vi "Configure Math Function (Low-pass).vi"(4 "Math Function Index (1: Math Function 1)":i32(ring)=1 items=["Math Function 1"=1, "Math Function 2"=2, "Math Function 3"=3, "Math Function 4"=4], 8 "error in (no error)":errorcluster, 10 "Low-Pass Frequency (1E+9)":dbl=1000000000.0, 11 "VISA resource name":refnum<visa-resource-name>) -> (0 "error out":errorcluster, 3 "VISA resource name out":refnum<visa-resource-name>)   [LabVIEW 2015, in "Agilent 2000 3000 X-Series.lvlib"]
doc: "Configures the low-pass math function.\n\n<B>Note(s):</B>\nThis function is available only with the DSOX3ADVMATH advanced math license."
uses:
  <instrlib>/Agilent 2000 3000 X-Series/Agilent 2000 3000 X-Series.lvlib
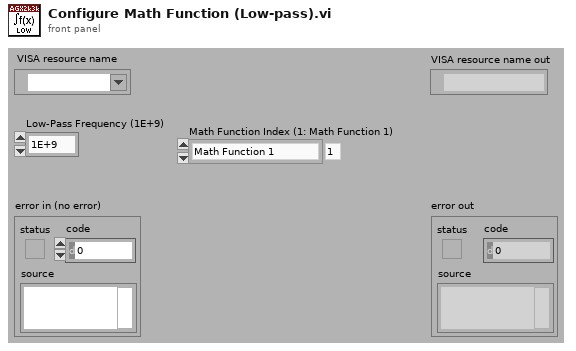
[diagram p1: front panel]
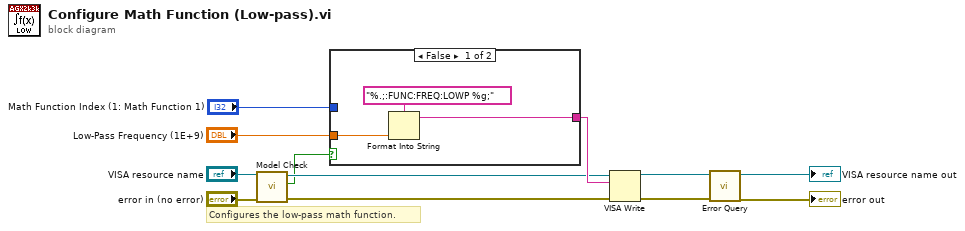
[diagram p0: block diagram]
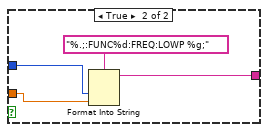
[diagram p2: hidden frame]
diagram:
  # "Configures the low-pass math function."
  n1 = call <instrlib>:"Model Check.vi"("error in (no error)"="error in (no error)", "VISA resource name"="VISA resource name") -> ("error out"=w3:errorcluster, "Not 2000 or 3000 Series"=w2:bool, "VISA resource name out"=w4:refnum<visa-resource-name>)  [unwired: 7 out]
  n2 = case shown="False" w2 {
    tunnel: "Low-Pass Frequency (1E+9)" -> [w14 w17]
    tunnel: [w13 w16] -> w11
    tunnel: "Math Function Index (1: Math Function 1)" -> [_ w18]
    frame False {
      n3 = Format Into String(format string="%.;:FUNC:FREQ:LOWP %g;", w14) -> (resulting string=w13:string)  [unwired: 2 in, 1 out]
    }
    frame True {
      n4 = Format Into String(format string="%.;:FUNC%d:FREQ:LOWP %g;", w18, w17) -> (resulting string=w16:string)  [unwired: 2 in, 1 out]
    }
  }
  n5 = VISA Write(VISA resource name=w4, write buffer=w11, error in (no error)=w3) -> (VISA resource name out=w10:refnum<visa-resource-name>, error out=w9:errorcluster)  [unwired: 1 out]
  n6 = call <instrlib>:"Error Query.vi"("error in (no error)"=w9, "VISA resource name"=w10) -> ("error out"=→"error out":errorcluster, "VISA resource name out"=→"VISA resource name out":refnum<visa-resource-name>)  [unwired: 8 out]
